vi "T7 Stream Logger KAG.vi"() -> ()   [LabVIEW 2022 SP3]
doc: "This VI is quickly devised to Run T7 Stream function at an adjustable / user-prescribed interval which is wired to the timeout value of an event structure containing the LJT7DAQ Acquisition Plugin VI. A couple of the VIs require modification. The Plugin Control Terminal has a file path input. The Byte to Volt.vi handles the data writing."
panel:
  out "error out":errorcluster
  in  "stop":bool
  in  "Minutes between Logs":dbl
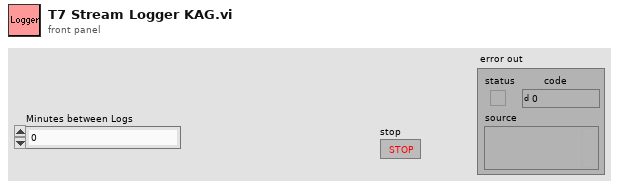
[diagram p1: front panel]
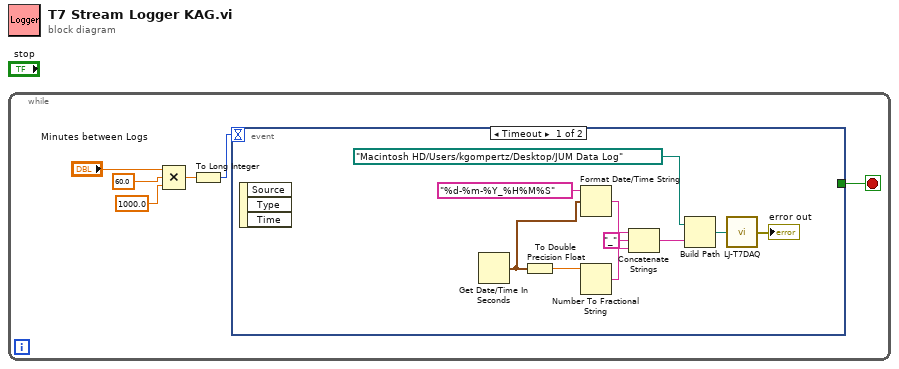
[diagram p0: block diagram]
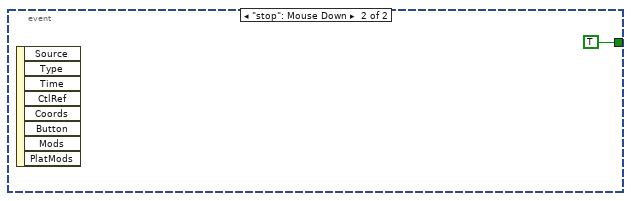
[diagram p2: hidden frame]
diagram:
  n1 = while {
    stop <- w2 stop-if-true
    n2 = Compound Arithmetic op=MULTIPLY("Minutes between Logs", 60.0 ("value"), 1000.0 ("value")) -> (w3:dbl)
    n3 = To Long Integer(number=w3) -> (32bit integer=w1:i32)
    n4 = event shown="[0] Timeout" {
      selector: _ -> [_ _]
      dyn-events: _ -> [_ _]
      timeout: w1 -> [_ _]
      tunnel: [_ TRUE] -> w2
      event Timeout {
        n5 = event-data() -> ()  [unwired: 1 in, 3 out]
        n6 = Get Date/Time In Seconds() -> (seconds since 1Jan1904=w13:timestamp)
        n7 = To Double Precision Float(number=w13) -> (double precision float=w12:dbl)
        n8 = Format Date/Time String(time format string (%c)="%d-%m-%Y_%H%M%S", seconds (now)=w13) -> (date/time string=w9:string)  [unwired: 1 in]
        n9 = Number To Fractional String(number=w12) -> (F-format string=w10:string)  [unwired: 3 in]
        n10 = Concatenate Strings(w9, "_" ("string"), w10) -> (w8:string)
        n11 = Build Path(base path=path "/Macintosh HD/Users/kgompertz/Desktop/JUM Data Log" ("Destination Path"), name or relative path=w8) -> (appended path=w15:path)
        n12 = call "LJ-T7DAQ.vi"(1:w15) -> ("Error Out"=→"error out":errorcluster)
      }
      event "stop": Mouse Down {
        n13 = event-data() -> ()  [unwired: 1 in, 8 out]
      }
    }
  }
